vi "SetCurrent(Advanced).vi"(5 "Step":i8=1 min=1 max=24, 7 "Memory":i8=1 min=1 max=50, 8 "Error In":errorcluster, 10 "Current":dbl min=0.0 max=10.0 format="%.2g", 11 "VISA resource name":refnum<visa-resource-name>) -> (0 "Error Out":errorcluster, 3 "VISA resource name out":refnum<visa-resource-name>)   [LabVIEW 2013]
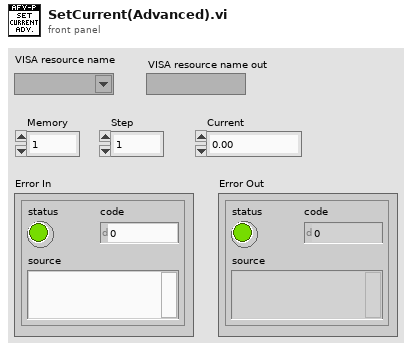
[diagram p1: front panel]
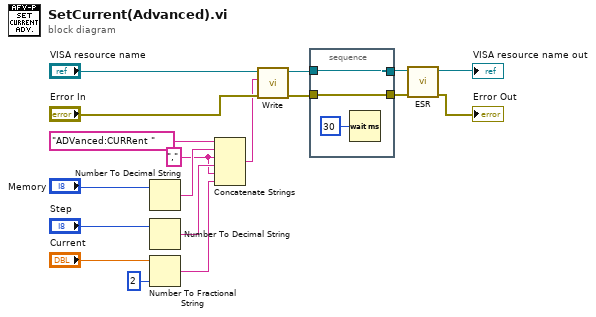
[diagram p0: block diagram]
diagram:
  w7 = "," ("string")
  n1 = Number To Decimal String(number="Memory") -> (decimal integer string=w11:string)  [unwired: 1 in]
  n2 = Number To Decimal String(number="Step") -> (decimal integer string=w8:string)  [unwired: 1 in]
  n3 = Number To Fractional String(number="Current", precision (6)=i16 2) -> (F-format string=w9:string)  [unwired: 2 in]
  n4 = Concatenate Strings("ADVanced:CURRent " ("Write Buffer"), w11, w7, w8, w7, w9) -> (w13:string)
  n5 = call "Write.vi"("Error In"="Error In", "Write Buffer"=w13, "VISA resource name"="VISA resource name") -> ("Error Out"=w3:errorcluster, "VISA resource name out"=w4:refnum<visa-resource-name>)  [unwired: 7 in]
  n6 = stacked-sequence {
    tunnel: [w20] -> w6
    tunnel: w4 -> [w20]
    tunnel: [w19] -> w5
    tunnel: w3 -> [w19]
    frame #0 {
      n7 = Wait (ms)(milliseconds to wait=u32 30) -> ()  [unwired: 1 out]
    }
  }
  n8 = call "ESR.vi"("Error In"=w5, "VISA resource name"=w6) -> ("Error Out"=→"Error Out":errorcluster, "VISA resource name out"=→"VISA resource name out":refnum<visa-resource-name>)  [unwired: 8 in]
